vi "Write Configure Tester.vi"(8 "error in (no error)":errorcluster, 10 "Configure Tester":T1, 11 "Potting Procedure in":refnum<class "Potting Procedure.lvclass">) -> (0 "error out":errorcluster, 3 "Potting Procedure out":refnum<class "Potting Procedure.lvclass">)   [LabVIEW 2011, in "Potting Procedure.lvclass"]
uses:
  Potting Procedure.lvclass
  Type Definitions/Configure Tester.ctl
  UI typedefs/Chuck Control.ctl
  UI typedefs/Chuck Slot Control.ctl
  Potting Procedure.lvclass/Potting Procedure.ctl
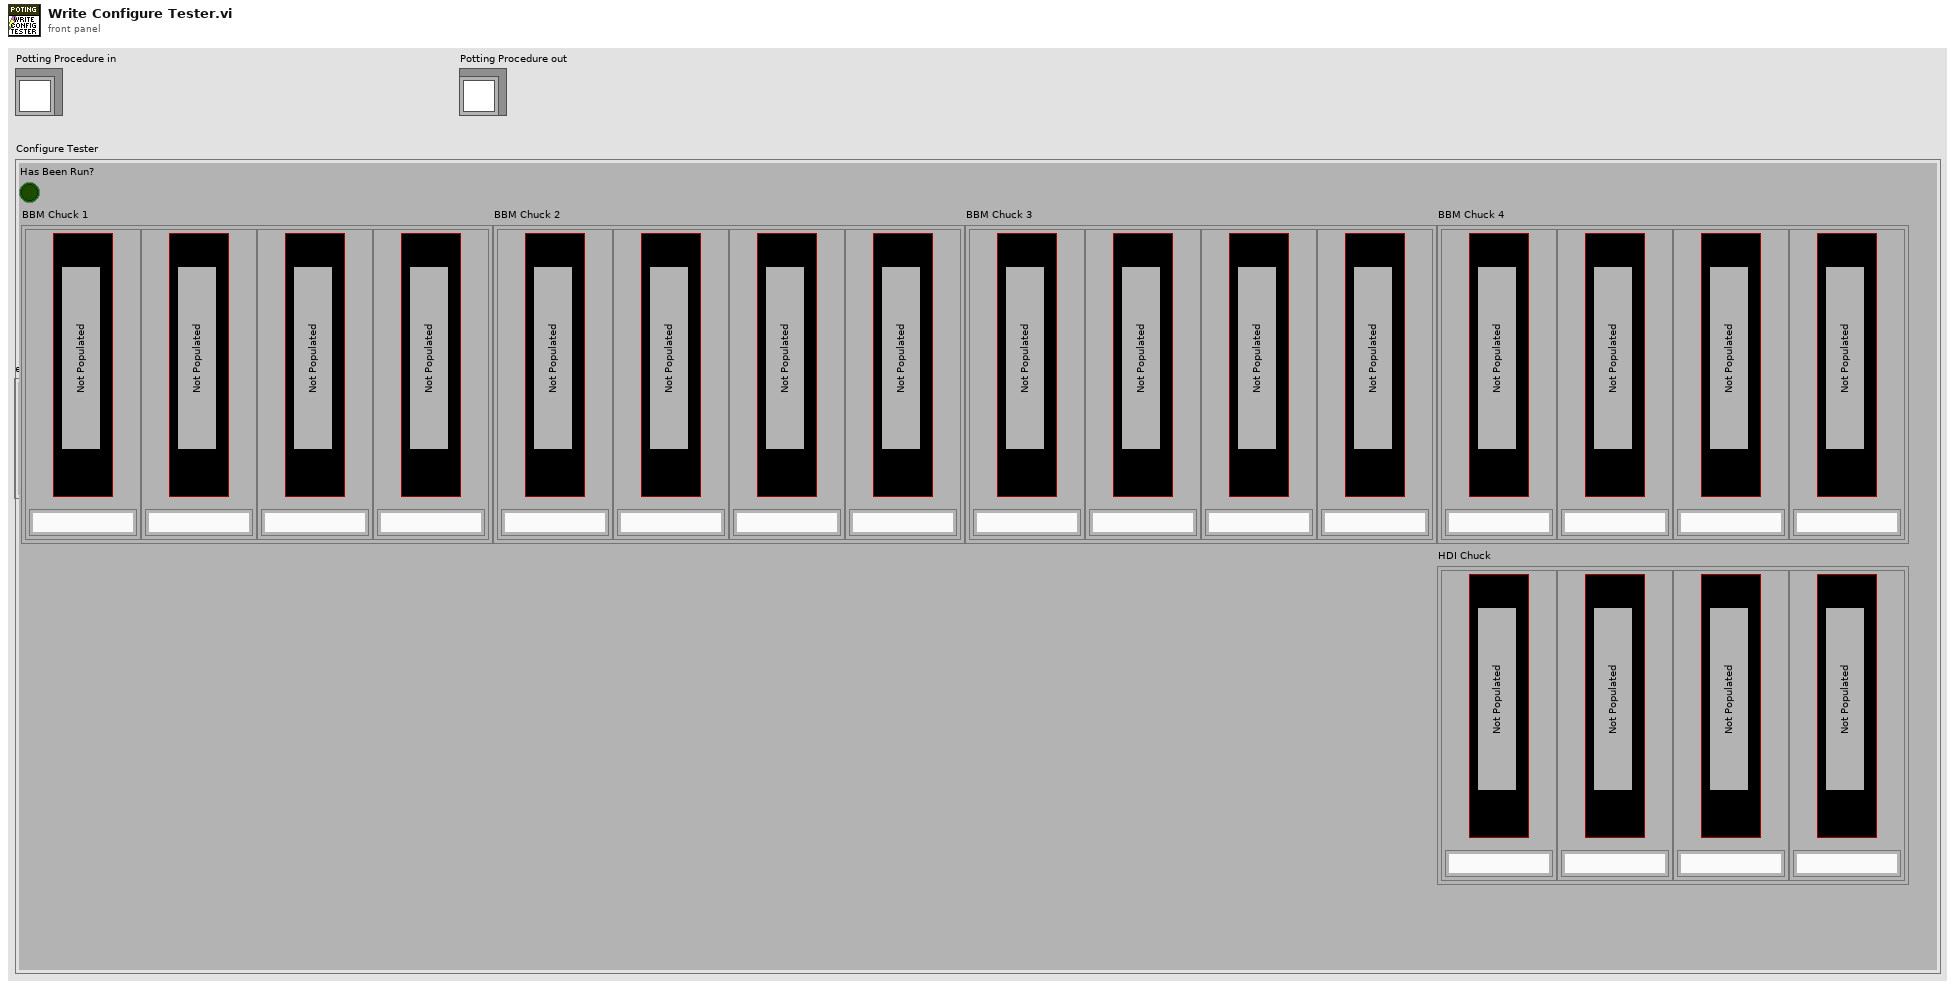
[diagram p1: front panel]
types:
  T1 = typedef "Configure Tester.ctl" = cluster{"Has Been Run?":bool, "BBM Chuck 1":T2, "BBM Chuck 2":T2, "BBM Chuck 3":T2, "BBM Chuck 4":T2, "HDI Chuck":T2}
  T2 = typedef "Chuck Control.ctl" = cluster{"Slot 1":T3, "Slot 2":T3, "Slot 3":T3, "Slot 4":T3}
  T3 = typedef "Chuck Slot Control.ctl" = cluster{"Slot Populated":bool, "S/N":string}
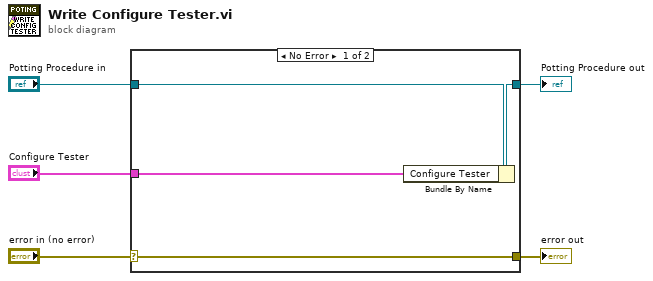
[diagram p0: block diagram]
diagram:
  n1 = case shown="No Error" "error in (no error)" {
    selector: "error in (no error)" -> [w9 w10]
    tunnel: [w9 w10] -> w4
    tunnel: [w7 w11] -> w2
    tunnel: "Potting Procedure in" -> [w8 w11]
    tunnel: "Configure Tester" -> [w6 _]
    frame No Error {
      n2 = Bundle By Name(cluster=w8, "Configure Tester"=w6) -> (w7:refnum<class "Potting Procedure.lvclass">)
    }
    frame Error {
    }
  }
  "error out" <- w4
  "Potting Procedure out" <- w2
